vi "Handle Power Switch.vi"(8 "error in":errorcluster, 10 "Power Setup":u8, 11 "Controller in":refnum<class "Controller.lvclass">) -> (0 "error out":errorcluster, 3 "Controller out":refnum<class "Controller.lvclass">)   [LabVIEW 2014, in "Controller.lvlib" / "Controller.lvclass"]
uses:
  Controller.lvclass
  SuperActor/SuperClass.lvclass/SuperClass.ctl
  SuperActor/Read CVT Session.vi
  SuperActor/Read Log Session.vi
  <vilib>/DAQmx/write.llb/DAQmx Write (Digital 1D Bool NChan 1Samp 1Line).vi
  <vilib>/DAQmx/write.llb/DAQmx Write (Digital Bool 1Line 1Point).vi
  <userlib>/_Session Fwk/Session - Root.lvclass
  reusable/Session APIs/Session Log/System Log.lvclass
  reusable/Session APIs/CVT/CVT.lvclass
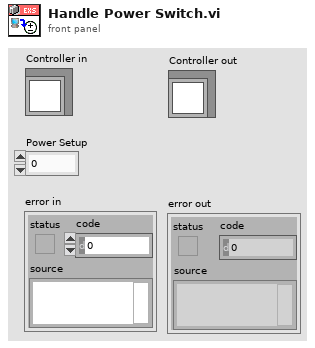
[diagram p1: front panel]
types:
  T1 = typedef "Session - Root.lvclass/Session Handle.ctl" = refnum<data-value>
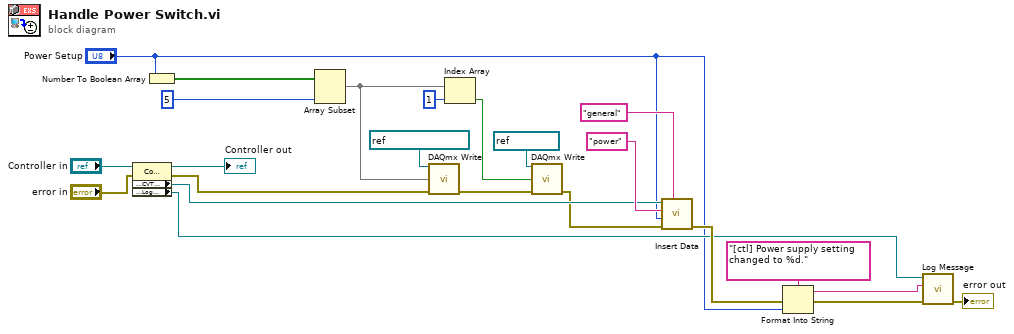
[diagram p0: block diagram]
diagram:
  n1 = property class="Controller"(reference="Controller in", error in="error in") -> (reference out=→"Controller out":refnum<class "Controller.lvclass">, error out=w16:errorcluster, "Accessors:CVT Session"=w8:T1, "Accessors:Log Session"=w9:T1)
  n2 = Number To Boolean Array(number="Power Setup") -> (Boolean array=w23:bool[])
  n3 = Array Subset(array=w23, length=5) -> (w13:bool[])  [unwired: 1 in]
  n4 = call-poly <vilib>:"DAQmx Write.vi"("task/channels in"=refnum<k21> "Power Supply", "data"=w13, "error in"=w16) -> ("error out"=w7:errorcluster)  [unwired: 10 in, 2 out]
  n5 = Index Array(array=w13, index=1) -> (element=w10:bool)
  n6 = call-poly <vilib>:"DAQmx Write.vi"("task/channels in"=refnum<k21> "O3 LED", "data"=w10, "error in"=w7) -> ("error out"=w6:errorcluster)  [unwired: 10 in, 2 out]
  n7 = call "Insert Data.vi"("Group"="general", "error in"=w6, "Data"="Power Setup", "tag"="power", "CVT Session In"=w8) -> ("error out"=w15:errorcluster)  [unwired: 5 in, 1 out]
  n8 = Format Into String(format string="[ctl] Power supply setting changed to %d.", error in=w15, "Power Setup") -> (resulting string=w19:string, error out=w14:errorcluster)  [unwired: 1 in]
  n9 = call "Log Message.vi"("error in"=w14, "MSG In"=w19, "session in"=w9) -> ("error out"=→"error out":errorcluster)  [unwired: 7 in, 1 out]
